vi "Read Value.vi"(8 "error in (no error)":errorcluster caption="entrée d'erreur (pas d'erreur)", 11 "DAQmxTaskAITension en entrée":refnum<class "DAQmxTaskAIVoltage.lvclass">) -> (0 "error out":errorcluster caption="sortie d'erreur", 1 "Data":bool, 2 "Data string":string, 3 "DAQmxTaskAITension en sortie":refnum<class "DAQmxTaskAIVoltage.lvclass">)   [LabVIEW 2015, in "DAQmxTaskAIVoltage.lvclass"]
uses:
  DAQmxTaskAIVoltage.lvclass
  DAQmxTask.lvclass/DAQmxTask.ctl
  <vilib>/DAQmx/read.llb/DAQmx Read (Analog 1D DBL NChan 1Samp).vi
  <vilib>/DAQmx/miscellaneous.llb/DAQmx Fill In Error Info.vi
  DAQmxTask.lvclass
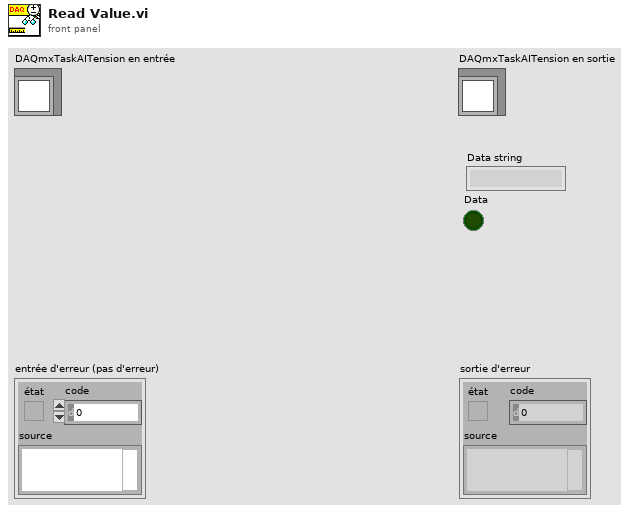
[diagram p1: front panel]
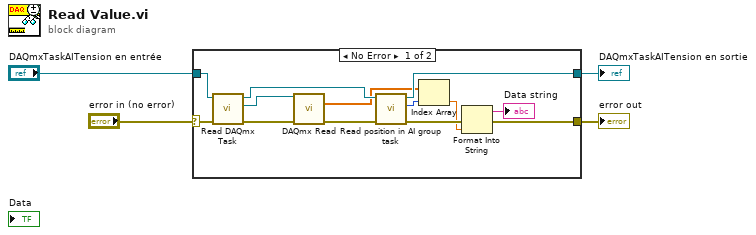
[diagram p0: block diagram]
diagram:
  n1 = case shown="No Error" "error in (no error)" {
    selector: "error in (no error)" -> [w17 w18]
    tunnel: [w8 w19] -> w2
    tunnel: "DAQmxTaskAITension en entrée" -> [w16 w19]
    tunnel: [w13 w18] -> w4
    frame No Error {
      n2 = call "Read DAQmx Task.vi"("error in (no error)"=w17, "DAQmxTask in"=w16) -> ("error out"=w15:errorcluster, "DAQmx Task Name"=w14:refnum<k21>, "DAQmxTask out"=w9:refnum<class "DAQmxTaskAIVoltage.lvclass">)  [unwired: 7 in]
      n3 = call-poly <vilib>:"DAQmx Read.vi"("task/channels in"=w14, "error in"=w15) -> ("data"=w6:dbl[], "error out"=w11:errorcluster)  [unwired: 11 in, 1 out]
      n4 = call "Read position in AI group task.vi"("error in (no error)"=w11, "DAQmxTask in"=w9) -> ("error out"=w10:errorcluster, "position in AI group task"=w7:i32, "DAQmxTask out"=w8:refnum<class "DAQmxTaskAIVoltage.lvclass">)  [unwired: 7 in]
      n5 = Index Array(array=w6, index=w7) -> (element=w5:dbl)
      n6 = Format Into String(error in=w10, w5) -> (resulting string=→"Data string":string, error out=w13:errorcluster)  [unwired: 2 in]
    }
    frame Error {
    }
  }
  "error out" <- w4
  "DAQmxTaskAITension en sortie" <- w2
